vi "SetupSoundParams.vi"(2 "error in (no error)":errorcluster, 3 "#Channels":refnum<vi>, 4 "Sample Rate (Hz)":refnum<vi>, 5 "device":u32) -> (0 "error out":errorcluster, 1 "device out":u32)   [LabVIEW 2014]
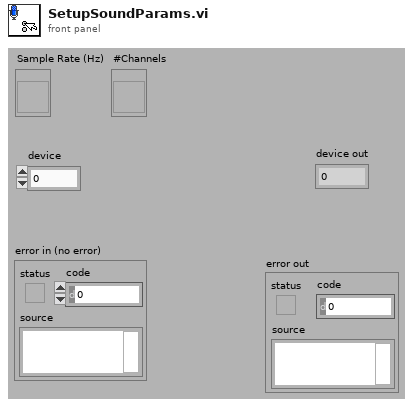
[diagram p1: front panel]
types:
  T1 = cluster{"channels":i32[], "depths":i32[], "minFreq":dbl, "maxFreq":dbl}
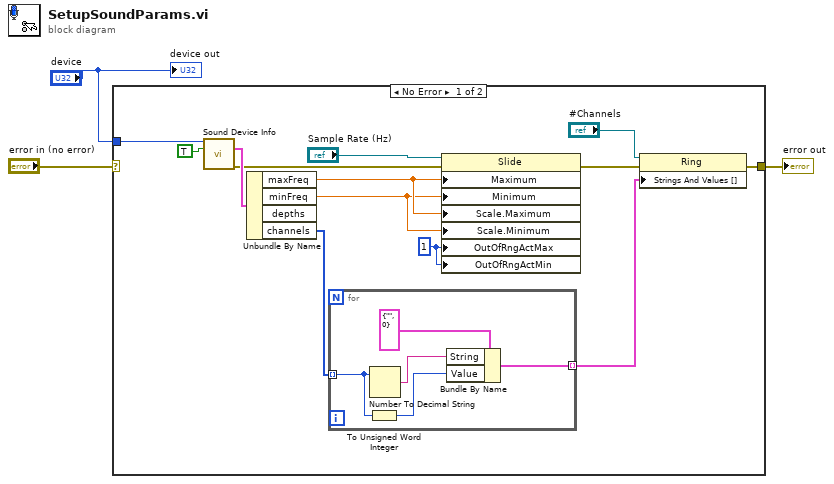
[diagram p0: block diagram]
diagram:
  n1 = case shown="No Error" "error in (no error)" {
    selector: "error in (no error)" -> [_ w22]
    tunnel: [w9 w22] -> w3
    tunnel: "device" -> [w4 _]
    frame No Error {
      w6 = u8 1 ("Out Of Range Action:Maximum")
      n2 = call <vilib>:"Sound Device Info.vi"("device"=w4, "isInput?"=TRUE) -> ("Capabilities"=w15:T1, "error out"=w12:errorcluster)  [unwired: 1 in, 11 out]
      n3 = Unbundle By Name(w15) -> ("maxFreq"=w8:dbl, "minFreq"=w7:dbl, "channels"=w13:i32[])  [unwired: 1 out]
      n4 = for {
        tunnel: w13 -> [w21] mode=indexing
        tunnel: [w18] -> w10 mode=indexing
        n5 = To Unsigned Word Integer(number=w21) -> (unsigned 16bit integer=w17:u16)
        n6 = Number To Decimal String(number=w21) -> (decimal integer string=w19:string)  [unwired: 1 out]
        n7 = Bundle By Name(cluster=cluster{"String":string, "Value":u16} {"String"="", "Value"=0}, "String"=w19, "Value"=w17) -> (w18:cluster{"String":string, "Value":u16})
      }
      n8 = property class="Slide"(reference="Sample Rate (Hz)", error in=w12, "Maximum"=w8, "Minimum"=w7, "Scale.Maximum"=w8, "Scale.Minimum"=w7, "OutOfRngActMax"=w6, "OutOfRngActMin"=w6) -> (error out=w5:errorcluster)  [unwired: 1 out]
      n9 = property class="Ring"(reference="#Channels", error in=w5, "Strings And Values []"=w10) -> (error out=w9:errorcluster)  [unwired: 1 out]
    }
    frame Error {
    }
  }
  "error out" <- w3
  "device out" <- "device"
